vi "Add Current Aircraft Pos to Route.vi"(8 "Error In":errorcluster) -> (0 "Error Out":errorcluster)   [LabVIEW 2014]
uses:
  C:/Robotic Systems/Products/AgFalcon/Software/Ground Station/Data/Mapping DLL/GMap.NET.Core.dll
  Data/Mapping DLL/GMap.NET.Core.dll
  Aircraft Information/Sub VI/Selected Aircraft/SubVI/Get Selected Aircraft.vi
  Aircraft Information/Sub VI/Get Aircraft GPS.vi
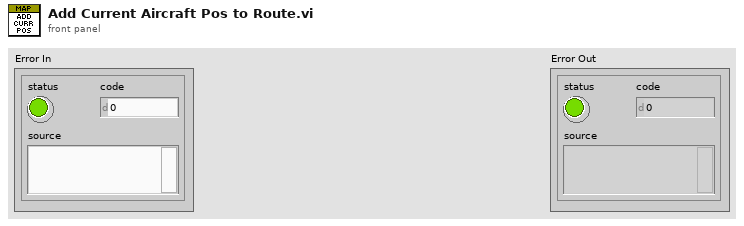
[diagram p1: front panel]
types:
  T1 = typedef "Aircraft GPS Data.ctl" = cluster{"Latitude (degrees)":dbl, "Longitude (degrees)":dbl, "Altitude (m)":dbl, "Fix Type":u8, "HDOP (cm)":u16, "VDOP (cm)":u16, "Ground Speed (m/s)":dbl, "Coarse Over Ground (degrees)":u16, "Number of Satellites":u8}
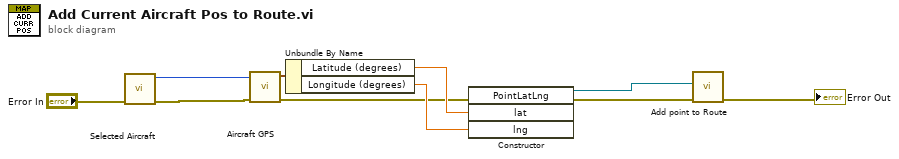
[diagram p0: block diagram]
diagram:
  n1 = call-poly "Selected Aircraft.vi"("Error In"="Error In") -> ("Error Out"=w10:errorcluster, "Selected Aircraft ID Out"=w9:u8)  [unwired: 9 in]
  n2 = call-poly "Aircraft GPS.vi"("Error In"=w10, "Aircraft ID"=w9) -> ("Error Out"=w1:errorcluster, "Aircraft GPS Data Out"=w8:T1)  [unwired: 8 in]
  n3 = Unbundle By Name(w8) -> ("Latitude (degrees)"=w7:dbl, "Longitude (degrees)"=w6:dbl)
  n4 = constructor class="PointLatLng"(error in=w1, "lat"=w7, "lng"=w6) -> (reference out=w5:refnum<k24>, error out=w2:errorcluster)  [unwired: 2 in, 3 out]
  n5 = call "Add point to Route.vi"("Error In"=w2, "New Point"=w5) -> ("Error Out"=→"Error Out":errorcluster)  [unwired: 9 in]
